vi "setParallelSpeed.vi"(6 "Delay between send and receive [ms]":i32=1000, 8 "error in (no error)":errorcluster, 10 "token":i32, 11 "CCD in":refnum<class "CCD.lvclass">) -> (0 "error out":errorcluster, 1 "ID":i32, 2 "results-JSON string":string, 3 "CCD out":refnum<class "CCD.lvclass">)   [LabVIEW 2023, in "CCD.lvclass"]
doc: "Sets the CCD parallel speed token. A list of supported parallel speed tokens can be found in the CCD configuration. See ccd_getConfig command.\n\nNote: The Parallel Speed value may also be referred to as the Vertical Shift Rate. These terms are interchangeable.\n\nFor example:\n\n\"parallelSpeeds\": [\n {\n \"info\": \"9.6 µSec\",\n \"token\": 1\n },\n {\n \"info\": \"4.9 µSec\",\n \"token\": 2\n },\n {\n \"info\": \"19 µSec\",\n \"token\": 0\n }\n],"
uses:
  CCD.lvclass
  CCD.lvclass/CCD.ctl
  20f7d3bd-08ac-4524-9bed-df36c1da25a0.vi
  GenericDevice/GenericDevice.lvclass
  cab240a6-cbf4-4e2c-ab79-96d9c1b88265.vi
panel:
  # "Connector Pane"
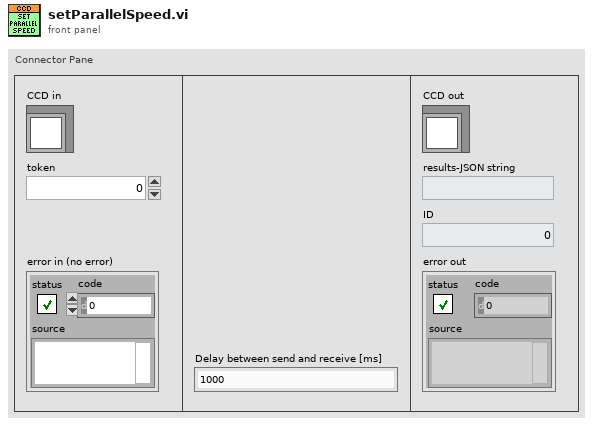
[diagram p1: front panel]
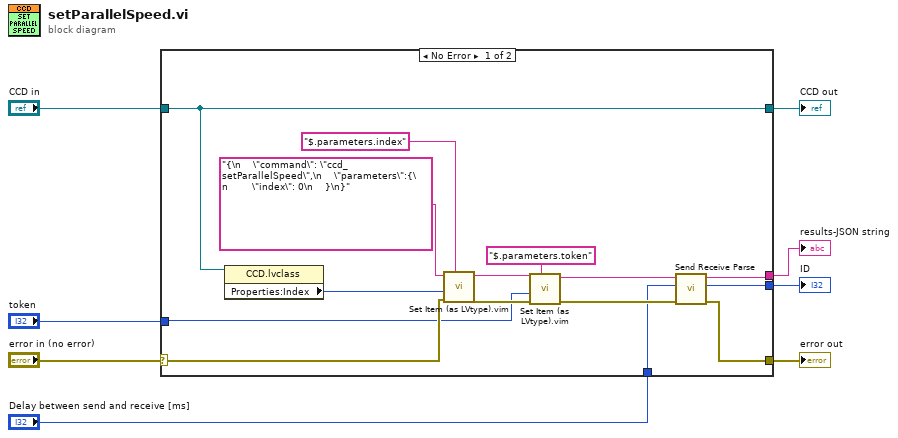
[diagram p0: block diagram]
diagram:
  n1 = case shown="No Error" "error in (no error)" {
    selector: "error in (no error)" -> [w19 w25]
    tunnel: [w14 w25] -> w7
    tunnel: [w21 w24] -> w5
    tunnel: "CCD in" -> [w21 w24]
    tunnel: [w13 _] -> w4
    tunnel: [w12 _] -> w3
    tunnel: "Delay between send and receive [ms]" -> [w10 _]
    tunnel: "token" -> [w9 _]
    frame No Error {
      n2 = property class="CCD.lvclass"(reference=w21) -> ("Properties:Index"=w20:i32)  [unwired: 1 in, 2 out]
      n3 = call "Set Item (as LVtype).vim"("$Path or Item Name"="$.parameters.index", "error in (no error)"=w19, "Anything"=w20, "JSON"="{\n    \"command\": \"ccd_setParallelSpeed\",\n    \"parameters\":{\n        \"index\": 0\n    }\n}") -> ("error out"=w17:errorcluster, "<JSON>"=w15:string)  [unwired: 4 in, 1 out]
      n4 = call "Set Item (as LVtype).vim"("$Path or Item Name"="$.parameters.token", "error in (no error)"=w17, "Anything"=w9, "JSON"=w15) -> ("error out"=w16:errorcluster, "<JSON>"=w11:string)  [unwired: 4 in, 1 out]
      n5 = call "Send Receive Parse.vi"("error in"=w16, "Delay between send and receive [ms]"=w10, "<JSON>"=w11) -> ("error out"=w14:errorcluster, "ID"=w12:i32, "results-JSON string"=w13:string)  [unwired: 6 in]
    }
    frame Error {
    }
  }
  "error out" <- w7
  "CCD out" <- w5
  "results-JSON string" <- w4
  "ID" <- w3
